vi "Write Running TS.vi"(8 "error in (no error)":errorcluster, 11 "CIFCorePlugin in":refnum<class "CIFCorePlugin.lvclass">) -> (0 "error out":errorcluster, 3 "CIFCorePlugin out":refnum<class "CIFCorePlugin.lvclass">)   [LabVIEW 2021, in "CIFCorePlugin.lvclass"]
doc: "Update the timestamp. Time is U64, absolute time in nS in the appropriate clockID configured for the plugin. If a 0 is wired it will automatically get the current time."
uses:
  CIFCorePlugin.lvclass
  CIFCorePlugin.lvclass/CIFCorePlugin.ctl
  CIFUtilities/CIFClocks/Typedef/Future Time Event Limits.ctl
  CIFUtilities/CIFClocks/Time Conversion/LabVIEW Time to UTC Time.vi
  CIFUtilities/CIFClocks/SubVIs/Add Error.vi
  CIFUtilities/CIFClocks/CIFClocks.lvlib
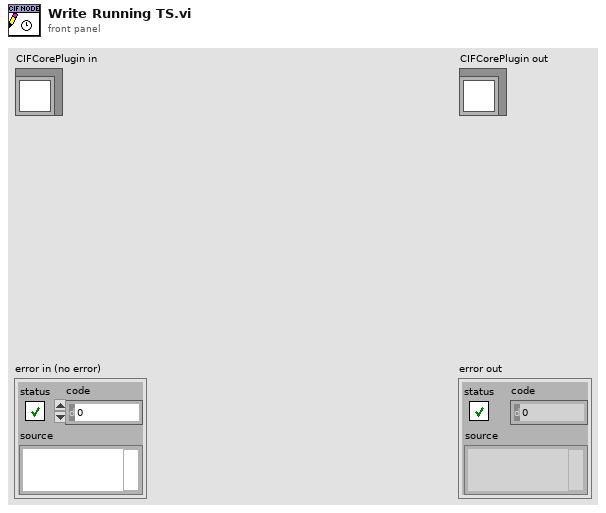
[diagram p1: front panel]
types:
  T1 = typedef "CIFClocks.lvlib/Future Time Event Limits.ctl" = cluster{"Maximum":u64, "Minimum":u64}
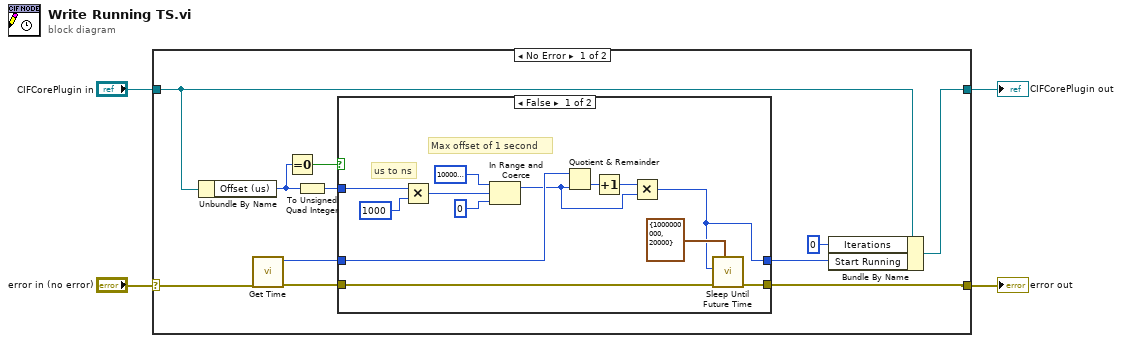
[diagram p0: block diagram]
diagram:
  n1 = case shown="No Error" "error in (no error)" {
    selector: "error in (no error)" -> [w13 w31]
    tunnel: [w6 w31] -> w3
    tunnel: [w15 w32] -> w1
    tunnel: "CIFCorePlugin in" -> [w14 w32]
    frame No Error {
      n2 = Unbundle By Name(w14) -> ("Offset (us)"=w9:i32)
      n3 = call "Get Time.vi"("error in (no error)"=w13) -> ("error out"=w7:errorcluster, "Time (ns)"=w12:u64)  [unwired: 8 in, 1 out]
      n4 = Equal To 0?(x=w9) -> (x = 0?=w10:bool)
      n5 = To Unsigned Quad Integer(1:w9) -> (0:w8:u64)
      n6 = case shown="False" w10 {
        tunnel: w12 -> [w26 w30]
        tunnel: [w16 w30] -> w11
        tunnel: w8 -> [w22 _]
        tunnel: w7 -> [w24 w29]
        tunnel: [w23 w29] -> w6
        frame False {
          # "us to ns"
          # "Max offset of 1 second"
          n7 = Multiply(x=w22, y=u64 1000) -> (x*y=w20:u64)
          n8 = In Range and Coerce(upper limit=u64 1000000000, x=w20, lower limit=u64 0) -> (coerced(x)=w17:u64)  [unwired: 1 out]
          n9 = Quotient & Remainder(x=w26, y=w17) -> (floor(x/y)=w19:u64)  [unwired: 1 out]
          n10 = Increment(x=w19) -> (x+1=w18:u64)
          n11 = Multiply(x=w18, y=w17) -> (x*y=w16:u64)
          n12 = call "Sleep Until Future Time.vi"("FTE Limits (ns)"=T1 {"Maximum"=1000000000, "Minimum"=20000}, "error in (no error)"=w24, "Wake Time"=w16) -> ("error out"=w23:errorcluster)  [unwired: 8 in]
        }
        frame True {
        }
      }
      n13 = Bundle By Name(cluster=w14, "Iterations"=i64 0, "Start Running"=w11) -> (w15:refnum<class "CIFCorePlugin.lvclass">)
    }
    frame Error {
    }
  }
  "error out" <- w3
  "CIFCorePlugin out" <- w1
